vi "HFRR ADV v04 new software.vi"() -> ()   [LabVIEW 2025] (continued)
                n1292 = local write "FF 2"(0.0 ("FF 2")) -> ()
                n1293 = local write "reinit"(TRUE ("reinit")) -> ()
              }
            }
            n1294 = Select(t=0.0, s=w1593, f=w1592) -> (s? t:f=w1583:dbl)
            "COF 2" <- w1583
            n1295 = local write "COF 3"(w1583) -> ()
          }
        }
      }
    }
    n1296 = Wait (ms)(milliseconds to wait=u32 50) -> ()  [unwired: 1 out]
    n1297 = local read "Quit"() -> (w1521:bool)
    "Rate" <- 2500.0 ("No of Samples")
  }
  n1298 = while {
    tunnel: w57 -> [_]
    tunnel: [w1633] -> _
    tunnel: [w1609] -> w56
    i -> [w1633]
    stop <- w1609 stop-if-true
    # "C:\\LAB-IQ-NXT\\Scar View.exe"
    n1299 = local read "OK Button 16"() -> (w1622:bool)
    n1300 = local read "Main Tab"() -> (w1615:T2)
    n1301 = local read "service 3"() -> (w1616:bool)
    n1302 = local read "OPEN 6"() -> (w1618:bool)
    n1303 = local read "EDIT 2"() -> (w1620:bool)
    n1304 = flat-sequence {
      frame #0 {
        n1305 = local read "SAVE 2"() -> (w2235:bool)
        n1306 = stacked-sequence {
          frame #0 {
            n1307 = local read "EDIT"() -> (w2289:bool)
            n1308 = case shown="True" w2289 {
              tunnel: [u8 2 ("Disabled") u8 0 ("Disabled")] -> _
              frame False {
                w2291 = FALSE
                n1309 = local write "Password"("") -> ()
                n1310 = property on="SrvM CP" class="Bool (strict)"("Visible"=w2291) -> ()  [unwired: 2 in, 2 out]
                n1311 = property on="message" class="Str"("Visible"=w2291) -> ()  [unwired: 2 in, 2 out]
                n1312 = local write "x = y?"(w2291) -> ()
                n1313 = property on="Password" class="Str"("Visible"=w2291) -> ()  [unwired: 2 in, 2 out]
                n1314 = property on="ENTER THE NEW PASSWORD" class="Str"("Visible"=w2291) -> ()  [unwired: 2 in, 2 out]
                n1315 = property on="ENTER CURRENT PASSWORD" class="Str"("Visible"=w2291) -> ()  [unwired: 2 in, 2 out]
                n1316 = local write "SrvM CP"(w2291) -> ()
              }
              frame True {
                w2294 = TRUE
                n1317 = property on="SrvM CP" class="Bool (strict)"("Visible"=w2294) -> ()  [unwired: 2 in, 2 out]
                n1318 = property on="Password" class="Str"("Visible"=w2294) -> ()  [unwired: 2 in, 2 out]
              }
            }
            "dipl pwd" <- "@143$\n" ("dipl pwd")
          }
          frame #1 {
            # "Gain password"
            n1319 = String To Byte Array(string="ENTER CURRENT PASSWORD") -> (unsigned byte array=w2299:u8[])
            n1320 = Search 1D Array(1D array=w2299, element=u8 10) -> (index of element=w2302:i32)  [unwired: 1 in]
            n1321 = Index Array(array=w2299, index=w2302) -> (element=w2298:u8)
            n1322 = Equal?(x=w2298, y=10) -> (x = y?=w2296:bool)
            n1323 = case shown="True" w2296 {
              frame False {
                n1324 = property on="ENTER THE NEW PASSWORD" class="Str"("Visible"=FALSE) -> ()  [unwired: 2 in, 2 out]
              }
              frame True {
                # "password"
                # "change password logic"
                n1325 = local read "ENTER CURRENT PASSWORD"() -> (w2315:string)
                n1326 = local read "dipl pwd"() -> (w2309:string)
                n1327 = String To Byte Array(string=w2315) -> (unsigned byte array=w2317:u8[])
                n1328 = String To Byte Array(string=w2309) -> (unsigned byte array=w2310:u8[])
                n1329 = Array Size(array=w2317) -> (size(s)=w2314:i32)
                n1330 = Array Size(array=w2310) -> (size(s)=w2312:i32)
                n1331 = for {
                  N: w2314 -> [_]
                  tunnel: w2317 -> [w2341]
                  tunnel: [w2339] -> w2318 mode=indexing
                  tunnel: w2314 -> [w2333]
                  i -> [w2334]
                  n1332 = Decrement(x=w2333) -> (x-1=w2331:i32)
                  n1333 = Equal?(x=w2334, y=w2331) -> (x = y?=w2332:bool)
                  n1334 = Index Array(array=w2341, index=w2334) -> (element=w2335:u8)
                  n1335 = Number To Decimal String(number=w2335) -> (decimal integer string=w2340:string)  [unwired: 1 in]
                  n1336 = Select(t="", s=w2332, f="\r") -> (s? t:f=w2337:string)
                  n1337 = Concatenate Strings(w2340, w2337) -> (w2339:string)
                }
                n1338 = for {
                  N: w2312 -> [_]
                  tunnel: w2310 -> [w2329]
                  tunnel: [w2327] -> w2311 mode=indexing
                  tunnel: w2312 -> [w2324]
                  i -> [w2325]
                  n1339 = Decrement(x=w2324) -> (x-1=w2323:i32)
                  n1340 = Equal?(x=w2325, y=w2323) -> (x = y?=w2322:bool)
                  n1341 = Index Array(array=w2329, index=w2325) -> (element=w2328:u8)
                  n1342 = Number To Decimal String(number=w2328) -> (decimal integer string=w2326:string)  [unwired: 1 in]
                  n1343 = Select(t="", s=w2322, f="\r") -> (s? t:f=w2319:string)
                  n1344 = Concatenate Strings(w2326, w2319) -> (w2327:string)
                }
                n1345 = local read "string"() -> (w2316:string)
                n1346 = Concatenate Strings(w2311) -> (w2305:string)
                n1347 = Concatenate Strings(w2316) -> (w2313:string)
                n1348 = Concatenate Strings(w2318) -> (w2306:string)
                n1349 = Equal?(x=w2306, y=w2313) -> (x = y?=w2308:bool)
                n1350 = Equal?(x=w2306, y=w2305) -> (x = y?=w2304:bool)
                n1351 = Or(x=w2308, y=w2304) -> (x .or. y?=w2307:bool)
                n1352 = case shown="True" w2307 {
                  frame False {
                  }
                  frame True {
                    n1353 = property on="ENTER THE NEW PASSWORD" class="Str"("Visible"=TRUE) -> ()  [unwired: 2 in, 2 out]
                  }
                }
              }
            }
          }
          frame #2 {
            n1354 = String To Byte Array(string="ENTER THE NEW PASSWORD") -> (unsigned byte array=w2344:u8[])
            n1355 = Search 1D Array(1D array=w2344, element=u8 10) -> (index of element=w2348:i32)  [unwired: 1 in]
            n1356 = Index Array(array=w2344, index=w2348) -> (element=w2346:u8)
            n1357 = Equal?(x=w2346, y=10) -> (x = y?=w2343:bool)
            n1358 = case shown="False" w2343 {
              frame False {
              }
              frame True {
                n1359 = local write "EDIT"(FALSE) -> ()
                n1360 = local write "SrvM CP"(FALSE) -> ()
                n1361 = local read "ENTER THE NEW PASSWORD"() -> (w2351:string)
                n1362 = String To Byte Array(string=w2351) -> (unsigned byte array=w2356:u8[])
                n1363 = Array Size(array=w2356) -> (size(s)=w2353:i32)
                n1364 = for {
                  N: w2353 -> [_]
                  tunnel: w2356 -> [w2369]
                  tunnel: [w2366] -> w2358 mode=indexing
                  tunnel: w2353 -> [w2361]
                  i -> [w2359]
                  n1365 = Decrement(x=w2361) -> (x-1=w2362:i32)
                  n1366 = Equal?(x=w2359, y=w2362) -> (x = y?=w2363:bool)
                  n1367 = Index Array(array=w2369, index=w2359) -> (element=w2368:u8)
                  n1368 = Number To Decimal String(number=w2368) -> (decimal integer string=w2367:string)  [unwired: 1 in]
                  n1369 = Select(t="", s=w2363, f="\r") -> (s? t:f=w2360:string)
                  n1370 = Concatenate Strings(w2367, w2360) -> (w2366:string)
                }
                n1371 = local read "file path"() -> (w2350:path)
                n1372 = Concatenate Strings(w2358) -> (w2352:string)
                n1373 = Delete(path (use dialog)=w2350) -> (deleted path=w2354:path)  [unwired: 4 in, 2 out]
                n1374 = call <vilib>:"Write Characters To File.vi"("append to file? (new file:F)"=FALSE, "character string"=w2352, "file path (dialog if empty)"=w2354) -> ()  [unwired: 2 in, 1 out]
              }
            }
          }
          frame #3 {
            n1375 = case shown="True" "SrvM CP" {
              frame False {
                w2372 = ""
                n1376 = local write "ENTER CURRENT PASSWORD"(w2372) -> ()
                n1377 = local write "ENTER THE NEW PASSWORD"(w2372) -> ()
                n1378 = property on="ENTER CURRENT PASSWORD" class="Str"("Visible"=FALSE) -> ()  [unwired: 2 in, 2 out]
              }
              frame True {
                n1379 = property on="ENTER THE NEW PASSWORD" class="Str"() -> ("Visible"=w2373:bool)  [unwired: 2 in, 2 out]
                n1380 = Not(x=w2373) -> (.not. x?=w2374:bool)
                n1381 = property on="ENTER CURRENT PASSWORD" class="Str"("Visible"=w2374) -> ()  [unwired: 2 in, 2 out]
              }
            }
          }
          frame #4 {
            n1382 = String To Byte Array(string="Password") -> (unsigned byte array=w2381:u8[])
            n1383 = Search 1D Array(1D array=w2381, element=u8 10) -> (index of element=w2379:i32)  [unwired: 1 in]
            n1384 = Index Array(array=w2381, index=w2379) -> (element=w2380:u8)
            n1385 = Equal?(x=w2380, y=10) -> (x = y?=w2376:bool)
            n1386 = case shown="True" w2376 {
              frame False {
              }
              frame True {
                # "password"
                # "password"
                n1387 = local read "Password"() -> (w2394:string)
                n1388 = String To Byte Array(string=w2394) -> (unsigned byte array=w2397:u8[])
                n1389 = String To Byte Array(string="@143$\n") -> (unsigned byte array=w2383:u8[])
                n1390 = Array Size(array=w2397) -> (size(s)=w2392:i32)
                n1391 = Array Size(array=w2383) -> (size(s)=w2388:i32)
                n1392 = for {
                  N: w2392 -> [_]
                  tunnel: w2397 -> [w2431]
                  tunnel: [w2429] -> w2398 mode=indexing
                  tunnel: w2392 -> [w2426]
                  i -> [w2427]
                  n1393 = Decrement(x=w2426) -> (x-1=w2425:i32)
                  n1394 = Index Array(array=w2431, index=w2427) -> (element=w2430:u8)
                  n1395 = Equal?(x=w2427, y=w2425) -> (x = y?=w2424:bool)
                  n1396 = Number To Decimal String(number=w2430) -> (decimal integer string=w2428:string)  [unwired: 1 in]
                  n1397 = Select(t="", s=w2424, f="\r") -> (s? t:f=w2421:string)
                  n1398 = Concatenate Strings(w2428, w2421) -> (w2429:string)
                }
                n1399 = for {
                  N: w2388 -> [_]
                  tunnel: w2383 -> [w2442]
                  tunnel: [w2440] -> w2386 mode=indexing
                  tunnel: w2388 -> [w2437]
                  i -> [w2438]
                  n1400 = Decrement(x=w2437) -> (x-1=w2436:i32)
                  n1401 = Index Array(array=w2442, index=w2438) -> (element=w2441:u8)
                  n1402 = Equal?(x=w2438, y=w2436) -> (x = y?=w2435:bool)
                  n1403 = Number To Decimal String(number=w2441) -> (decimal integer string=w2439:string)  [unwired: 1 in]
                  n1404 = Select(t="", s=w2435, f="\r") -> (s? t:f=w2432:string)
                  n1405 = Concatenate Strings(w2439, w2432) -> (w2440:string)
                }
                n1406 = local read "file path"() -> (w2382:path)
                n1407 = call <vilib>:"Read Characters From File.vi"("file path (dialog if empty)"=w2382) -> ("character string"=w2396:string)  [unwired: 5 in, 3 out]
                "string" <- w2396
                n1408 = flat-sequence {
                  tunnel: [w2399] -> w2393
                  frame #0 {
                    w2399 = ""
                    n1409 = local write "Password"(w2399) -> ()
                  }
                }
                n1410 = Concatenate Strings(w2386) -> (w2387:string)
                n1411 = Concatenate Strings(w2396) -> (w2395:string)
                n1412 = Concatenate Strings(w2398) -> (w2390:string)
                n1413 = Equal?(x=w2390, y=w2395) -> (x = y?=w2385:bool)
                n1414 = Equal?(x=w2390, y=w2387) -> (x = y?=w2391:bool)
                n1415 = Or(x=w2385, y=w2391) -> (x .or. y?=w2384:bool)
                "x = y?" <- w2384
                n1416 = case shown="True" w2384 {
                  selector: w2384 -> [w2401 _]
                  tunnel: w2393 -> [_ _]
                  frame False {
                    n1417 = And(x=w2401, y=TRUE ("Visible")) -> (x .and. y?=w2402:bool)
                    n1418 = property on="message" class="Str"("Visible"=w2402) -> ()  [unwired: 2 in, 2 out]
                  }
                  frame True {
                    n1419 = control-ref of="This VI"() -> (w2413:refnum<vi>)
                    n1420 = property class="VI"(reference=w2413) -> (reference out=w2404:refnum<vi>, error out=w2408:errorcluster, "Panel"=w2412:refnum<vi>)  [unwired: 1 in]
                    n1421 = property on="message" class="Str"("Visible"=FALSE) -> ()  [unwired: 2 in, 2 out]
                    n1422 = property class="Pnl"(reference=w2412, error in=w2408) -> (reference out=w2406:refnum<vi>, error out=w2409:errorcluster, "Panes[]"=w2411:refnum<vi>[])
                    n1423 = for {
                      tunnel: w2411 -> [w2420] mode=indexing
                      tunnel: T15."Always On" ("Horizontal Scrollbar Visibility") -> [w2419]
                      tunnel: w2409 -> [w2416]
                      tunnel: [w2415] -> w2407
                      n1424 = property class="Pane"(reference=w2420, error in=w2416, "HorizScrollbarVisibility"=w2419) -> (reference out=w2417:refnum<vi>, error out=w2418:errorcluster)
                      n1425 = Close Reference(reference=w2417, error in (no error)=w2418) -> (error out=w2415:errorcluster)
                    }
                    n1426 = Close Reference(reference=w2406, error in (no error)=w2407) -> (error out=w2405:errorcluster)
                    n1427 = Close Reference(reference=w2404, error in (no error)=w2405) -> (error out=→"error out 6":errorcluster)
                  }
                }
              }
            }
          }
        }
        n1428 = local read "x = y?"() -> (w2241:bool)
        n1429 = local read "HUMIDITY: 2"() -> (w2243:dbl)
        n1430 = local read "HUMIDITY:"() -> (w2242:dbl)
        n1431 = property on="Port 2 Error" class="Clust (strict)"("Visible"="EDIT") -> ()  [unwired: 2 in, 2 out]
        n1432 = property on="Port 1 Error" class="Clust (strict)"("Visible"="EDIT") -> ()  [unwired: 2 in, 2 out]
        n1433 = case shown="True" "SrvM CP 2" {
          frame False {
          }
          frame True {
            n1434 = local write "SrvM CP 2"(FALSE ("SrvM CP 2")) -> ()
            n1435 = local read "HUMIDITY: 2"() -> (w2282:dbl)
            n1436 = local read "TEMP INTERCEPT: 2"() -> (w2281:dbl)
            n1437 = local read "DISPLACEMENT : 4"() -> (w2285:dbl)
            n1438 = local read "TEMPERATURE : 2"() -> (w2284:dbl)
            n1439 = local read "STROKE GAIN : 2"() -> (w2286:dbl)
            n1440 = local read "FRIC. FORCE : 2"() -> (w2287:dbl)
            n1441 = local read "AIR TEMP INTERCEPT: 2"() -> (w2280:dbl)
            n1442 = local read "AIR TEMPERATURE : 2"() -> (w2283:dbl)
            n1443 = local write "HUMIDITY:"(w2282) -> ()
            n1444 = local write "AIR TEMP INTERCEPT:"(w2281) -> ()
            n1445 = local write "TEMPERATURE :"(w2284) -> ()
            n1446 = local write "FRIC. FORCE :"(w2287) -> ()
            n1447 = local write "STROKE GAIN :"(w2286) -> ()
            n1448 = local write "DISPLACEMENT :"(w2285) -> ()
            n1449 = local write "AIR TEMPERATURE :"(w2283) -> ()
            n1450 = local write "TEMP INTERCEPT:"(w2280) -> ()
          }
        }
        n1451 = Or(x="SAVE", y=w2235) -> (x .or. y?=w2236:bool)
        n1452 = And(x="EDIT", y=w2241) -> (x .and. y?=w2239:bool)
        n1453 = local read "DISPLACEMENT : 4"() -> (w2252:dbl)
        n1454 = local read "TEMPERATURE : 2"() -> (w2250:dbl)
        n1455 = local read "STROKE GAIN : 2"() -> (w2256:dbl)
        n1456 = local read "DISPLACEMENT :"() -> (w2251:dbl)
        n1457 = local read "FRIC. FORCE : 2"() -> (w2259:dbl)
        n1458 = local read "TEMPERATURE :"() -> (w2248:dbl)
        n1459 = local read "STROKE GAIN :"() -> (w2255:dbl)
        n1460 = local read "FRIC. FORCE :"() -> (w2258:dbl)
        n1461 = case shown="True" w2239 {
          tunnel: [u8 2 ("Disabled") u8 0 ("Disabled")] -> w2238
          tunnel: [w2603 TRUE ("Visible")] -> w2237
          frame False {
            w2603 = FALSE ("Visible")
            n1462 = local write "EDIT 2"(w2603) -> ()
          }
          frame True {
          }
        }
        n1463 = case shown="True" w2236 {
          frame False {
          }
          frame True {
            n1464 = stacked-sequence {
              seq-local: [w2451 _ _] -> [_ w2598 _]
              frame #0 {
                (unwired) i16 5 ("precision (6)")
                # "[CH1]    - FF\n[CH2]   - TEMPERATURE\n[CH3]    - Humidity\n[CH4]    - AIR TEMP\n[CH5]\\- Visa Uno\n[CH6] \\- Visa Due\n[CH7]  \\- file path\n[CH8]   - Displacement Gain\n[CHA]   - Stroke Gain\n[CHB]   - Stroke PID Gain\n[CHC]   -Language Selection\n[CHD]   -Power +\n[CHE]   -Power_\n[CHF]   -Heater\n[CHG]   -Humidity Wet\n[CHH]   -Humidity Dry\n[CHI]   -Integral Time"
                n1465 = local read "Language Selection"() -> (w2499:enum16{"English", "Russian"})
                n1466 = local read "CH-HUMIDITY WET"() -> (w2457:u16)
                n1467 = local read "CH-HUMIDITY DRY"() -> (w2454:u16)
                n1468 = local read "STROKE GAIN :"() -> (w2443:dbl)
                n1469 = local read "CH-POWER +"() -> (w2466:u16)
                n1470 = local read "CH-POWER -"() -> (w2463:u16)
                n1471 = local read "CH-HEATER"() -> (w2460:u16)
                n1472 = local read "AIR TEMPERATURE :"() -> (w2446:dbl)
                n1473 = local read "DISPLACEMENT :"() -> (w2444:dbl)
                n1474 = local read "TEMPERATURE :"() -> (w2447:dbl)
                n1475 = local read "FRIC. FORCE :"() -> (w2448:dbl)
                n1476 = local read "HUMIDITY:"() -> (w2445:dbl)
                n1477 = Path To String(path="File Path") -> (string=w2515:string)
                n1478 = Number To Fractional String(number=w2443, width (-)=i16 10 ("precision (6)"), precision (6)=i16 5) -> (F-format string=w2506:string)  [unwired: 1 in]
                n1479 = Number To Fractional String(number=w2499, width (-)=i16 10 ("precision (6)"), precision (6)=i16 5) -> (F-format string=w2495:string)  [unwired: 1 in]
                n1480 = Number To Fractional String(number=w2466, width (-)=i16 10 ("precision (6)"), precision (6)=i16 5) -> (F-format string=w2489:string)  [unwired: 1 in]
                n1481 = Number To Fractional String(number=w2463, width (-)=i16 10 ("precision (6)"), precision (6)=i16 5) -> (F-format string=w2486:string)  [unwired: 1 in]
                n1482 = Number To Fractional String(number=w2460, width (-)=i16 10 ("precision (6)"), precision (6)=i16 5) -> (F-format string=w2481:string)  [unwired: 1 in]
                n1483 = Number To Fractional String(number=w2457, width (-)=i16 10 ("precision (6)"), precision (6)=i16 5) -> (F-format string=w2478:string)  [unwired: 1 in]
                n1484 = Number To Fractional String(number=w2454, width (-)=i16 10 ("precision (6)"), precision (6)=i16 5) -> (F-format string=w2473:string)  [unwired: 1 in]
                n1485 = local read "Com Port 1"() -> (w2450:refnum<visa-resource-name>)
                n1486 = local read "Com Port 2"() -> (w2449:refnum<visa-resource-name>)
                n1487 = Concatenate Strings(w2515, "\\" ("string")) -> (w2514:string)
                n1488 = Number To Fractional String(number=w2448, width (-)=i16 10 ("precision (6)"), precision (6)=i16 5) -> (F-format string=w2547:string)  [unwired: 1 in]
                n1489 = Number To Fractional String(number=w2447, width (-)=i16 10 ("precision (6)"), precision (6)=i16 5) -> (F-format string=w2546:string)  [unwired: 1 in]
                n1490 = Number To Fractional String(number=w2445, width (-)=i16 10 ("precision (6)"), precision (6)=i16 5) -> (F-format string=w2540:string)  [unwired: 1 in]
                n1491 = Number To Fractional String(number=w2446, width (-)=i16 10 ("precision (6)"), precision (6)=i16 5) -> (F-format string=w2534:string)  [unwired: 1 in]
                n1492 = Number To Fractional String(number=w2444, width (-)=i16 10 ("precision (6)"), precision (6)=i16 5) -> (F-format string=w2507:string)  [unwired: 1 in]
                n1493 = Concatenate Strings("[CHA]" ("string"), w2506, "- Stroke Gain" ("string"), "\r") -> (w2500:string)
                n1494 = Concatenate Strings("[CHC]" ("string"), w2495, "-Language Selection" ("string"), "\r") -> (w2492:string)
                n1495 = Concatenate Strings("[CHD]" ("string"), w2489, "-Power +" ("string"), "\r") -> (w2471:string)
                n1496 = Concatenate Strings("[CHG]" ("string"), w2478, "-Humidity Wet" ("string"), "\r") -> (w2468:string)
                n1497 = Concatenate Strings("[CHH]" ("string"), w2473, "-Humidity Dry" ("string"), "\r") -> (w2467:string)
                n1498 = Concatenate Strings("[CH1]" ("string"), w2547, " - FF" ("string"), "\r") -> (w2545:string)
                n1499 = Concatenate Strings("[CH2]" ("string"), w2546, " - TEMPERATURE" ("string"), "\r") -> (w2544:string)
                n1500 = Concatenate Strings("[CH3]" ("string"), w2540, " - Humidity" ("string"), "\r") -> (w2537:string)
                n1501 = Concatenate Strings("[CH4]" ("string"), w2534, " - AIR TEMP" ("string"), "\r") -> (w2530:string)
                n1502 = Concatenate Strings("[CH5]" ("string"), w2450, "- Visa Uno" ("string"), "\r") -> (w2523:string)
                n1503 = Concatenate Strings("[CH6]" ("string"), w2449, "- Visa Due" ("string"), "\r") -> (w2518:string)
                n1504 = Concatenate Strings("[CH7]" ("string"), w2514, "- file path" ("string"), "\r") -> (w2517:string)
                n1505 = Concatenate Strings("[CH8]" ("string"), w2507, "- Displacement Gain" ("string"), "\r") -> (w2510:string)
                n1506 = Concatenate Strings("[CHE]" ("string"), w2486, "-Power_" ("string"), "\r") -> (w2470:string)
                n1507 = Concatenate Strings("[CHF]" ("string"), w2481, "-Heater" ("string"), "\r") -> (w2469:string)
                n1508 = Concatenate Strings(w2545, w2544, w2537, w2530, w2523, w2518, w2517, w2510, w2500, w2492, w2471, w2470, w2469, w2468, w2467) -> (w2451:string)
                "gain" <- w2451
              }
              frame #1 {
                n1509 = local read "Camera Port :"() -> (w2559:string)
                n1510 = local read "C3 :"() -> (w2567:refnum<visa-resource-name>)
                n1511 = local read "TEMP INTERCEPT:"() -> (w2568:dbl)
                n1512 = local read "AIR TEMP INTERCEPT:"() -> (w2569:dbl)
                n1513 = Concatenate Strings("[CH8]" ("string"), w2559, "- Visa Camera" ("string"), "\r") -> (w2558:string)
                n1514 = Concatenate Strings("[CH7]" ("string"), w2567, "- Visa Humidity" ("string"), "\r") -> (w2563:string)
                n1515 = Number To Fractional String(number=w2568, width (-)=i16 10 ("precision (6)"), precision (6)=i16 5) -> (F-format string=w2586:string)  [unwired: 1 in]
                n1516 = local read "Com Port 3"() -> (w2570:refnum<visa-resource-name>)
                n1517 = Number To Fractional String(number=w2569, width (-)=i16 10 ("precision (6)"), precision (6)=i16 5) -> (F-format string=w2593:string)  [unwired: 1 in]
                n1518 = Concatenate Strings("[CHK]" ("string"), w2586, "-TEMP INTERCEPT" ("string"), "\r") -> (w2582:string)
                n1519 = Concatenate Strings("[SNO]" ("string"), "S.NO", "-" ("string"), "\r") -> (w2578:string)
                n1520 = Concatenate Strings("[CHJ]" ("string"), w2593, "-AIR TEMP INTERCEPT" ("string"), "\r") -> (w2583:string)
                n1521 = Concatenate Strings("[CHL]" ("string"), w2570, "- Visa humid" ("string"), "\r") -> (w2573:string)
                n1522 = String To Path(string="C:\\LAB-IQ\\calibrate WO 2465.dcf") -> (path=w2571:path)
                n1523 = Concatenate Strings(w2598, w2583, w2582, w2578, w2573, w2563, w2558) -> (w2597:string)
                n1524 = call <vilib>:"Write Characters To File.vi"("append to file? (new file:F)"=FALSE, "character string"=w2597, "file path (dialog if empty)"=w2571) -> ()  [unwired: 2 in, 1 out]
              }
              frame #2 {
                n1525 = local write "Lan flag"(0.0 ("Lan flag")) -> ()
                n1526 = local write "conststatus"(0.0 ("rpm value : 2")) -> ()
                n1527 = local write "SAVE"(FALSE ("OK Button 14")) -> ()
                n1528 = local write "SAVE 2"(FALSE ("SAVE 2")) -> ()
              }
            }
          }
        }
        n1529 = Subtract(x=w2243, y=w2242) -> (x-y=w2244:dbl)
        n1530 = local read "AIR TEMPERATURE : 2"() -> (w2247:dbl)
        n1531 = local read "AIR TEMPERATURE :"() -> (w2246:dbl)
        n1532 = Divide(x=w2244, y=w2242) -> (x/y=w2266:dbl)
        n1533 = Subtract(x=w2259, y=w2258) -> (x-y=w2257:dbl)
        n1534 = Subtract(x=w2250, y=w2248) -> (x-y=w2249:dbl)
        n1535 = Subtract(x=w2256, y=w2255) -> (x-y=w2254:dbl)
        n1536 = Subtract(x=w2252, y=w2251) -> (x-y=w2253:dbl)
        n1537 = Subtract(x=w2247, y=w2246) -> (x-y=w2245:dbl)
        n1538 = Divide(x=w2257, y=w2258) -> (x/y=w2277:dbl)
        n1539 = Divide(x=w2249, y=w2248) -> (x/y=w2270:dbl)
        n1540 = Divide(x=w2254, y=w2255) -> (x/y=w2274:dbl)
        n1541 = Divide(x=w2253, y=w2251) -> (x/y=w2273:dbl)
        n1542 = Multiply(x=w2266, y=100.0) -> (x*y=→"HUMIDITY  Calibration Error":dbl)
        n1543 = Divide(x=w2245, y=w2246) -> (x/y=w2269:dbl)
        n1544 = Multiply(x=w2277, y=100.0) -> (x*y=→"FRIC. FORCE Calibration Error":dbl)
        n1545 = Multiply(x=w2270, y=100.0) -> (x*y=→"TEMPERATURE  Calibration Error":dbl)
        n1546 = Multiply(x=w2274, y=100.0) -> (x*y=→"STROKE Calibration Error":dbl)
        n1547 = Multiply(x=w2273, y=100.0) -> (x*y=→"DISPLACEMENT  Calibration Error":dbl)
        n1548 = property on="EDIT 2" class="Bool (strict)"("Visible"=w2237) -> ()  [unwired: 2 in, 2 out]
        n1549 = property on="SAVE" class="Bool (strict)"("Visible"=w2237) -> ()  [unwired: 2 in, 2 out]
        n1550 = property on="SrvM CP" class="Bool (strict)"("Disabled"=w2238) -> ()  [unwired: 2 in, 2 out]
        n1551 = property on="visa due" class="CmbBox"("Disabled"=w2238) -> ()  [unwired: 2 in, 2 out]
        n1552 = property on="File Path" class="Path"("Disabled"=w2238) -> ()  [unwired: 2 in, 2 out]
        n1553 = Multiply(x=w2269, y=100.0) -> (x*y=→"AIR TEMPERATURE  Calibration Error":dbl)
        n1554 = property on="Language Selection" class="Enum (strict)"("Visible"=w2237) -> ()  [unwired: 2 in, 2 out]
        n1555 = property on="Tab Control 7" class="TabCtl (strict)"("Disabled"=w2238) -> ()  [unwired: 2 in, 2 out]
        n1556 = property on="AIR TEMP INTERCEPT:" class="DigNum (strict)"("Disabled"=w2238) -> ()  [unwired: 2 in, 2 out]
        n1557 = property on="CH-POWER -" class="DigNum (strict)"("Disabled"=w2238) -> ()  [unwired: 2 in, 2 out]
        n1558 = property on="CH-POWER +" class="DigNum (strict)"("Disabled"=w2238) -> ()  [unwired: 2 in, 2 out]
        n1559 = property on="AIR TEMPERATURE :" class="DigNum (strict)"("Disabled"=w2238) -> ()  [unwired: 2 in, 2 out]
        n1560 = property on="STROKE GAIN :" class="DigNum (strict)"("Disabled"=w2238) -> ()  [unwired: 2 in, 2 out]
        n1561 = property on="SPEED OUT:" class="DigNum (strict)"("Disabled"=w2238) -> ()  [unwired: 2 in, 2 out]
        n1562 = property on="CH-HUMIDITY DRY" class="DigNum (strict)"("Disabled"=w2238) -> ()  [unwired: 2 in, 2 out]
        n1563 = property on="HUMIDITY:" class="DigNum (strict)"("Disabled"=w2238) -> ()  [unwired: 2 in, 2 out]
        n1564 = property on="CH-HUMIDITY WET" class="DigNum (strict)"("Disabled"=w2238) -> ()  [unwired: 2 in, 2 out]
        n1565 = property on="TEMPERATURE :" class="DigNum (strict)"("Disabled"=w2238) -> ()  [unwired: 2 in, 2 out]
        n1566 = property on="DISPLACEMENT :" class="DigNum (strict)"("Disabled"=w2238) -> ()  [unwired: 2 in, 2 out]
        n1567 = property on="CH-HEATER" class="DigNum (strict)"("Disabled"=w2238) -> ()  [unwired: 2 in, 2 out]
        n1568 = property on="TEMP INTERCEPT:" class="DigNum (strict)"("Disabled"=w2238) -> ()  [unwired: 2 in, 2 out]
        n1569 = property on="FRIC. FORCE :" class="DigNum (strict)"("Disabled"=w2238) -> ()  [unwired: 2 in, 2 out]
      }
    }
    n1570 = local read "RUN"() -> (w1632:bool)
    n1571 = local read "RUN"() -> (w1630:bool)
    n1572 = disable-structure shown="Disabled" {
      disable-tunnel: [w1647 _] -> w1613
      disable-tunnel: [w1646 _] -> w1611
      frame Disabled {
        n1573 = local read "Temperature before test"() -> (w1640:dbl)
        n1574 = local read "Temperature after test"() -> (w1653:dbl)
        n1575 = case shown="True" "Save Results" {
          frame False {
          }
          frame True {
            w1669 = "\r"
            n1576 = local write "Save Results"(FALSE ("OK Button 5")) -> ()
            n1577 = local read "Temperature before test"() -> (w1707:dbl)
            n1578 = local read "Temperature after test"() -> (w1709:dbl)
            n1579 = local read "Humidity before test"() -> (w1706:dbl)
            n1580 = local read "Humidity after test"() -> (w1708:dbl)
            n1581 = local read "WS1.4"() -> (w1713:dbl)
            n1582 = local read "AVP"() -> (w1711:dbl)
            n1583 = Number To Fractional String(number=w1713, width (-)=i16 6, precision (6)=i16 1) -> (F-format string=w1673:string)  [unwired: 1 in]
            n1584 = local read "MWSD"() -> (w1710:dbl)
            n1585 = local read "String"() -> (w1702:string)
            n1586 = local read "FILE"() -> (w1705:string)
            n1587 = local read "HCF"() -> (w1712:dbl)
            n1588 = Number To Fractional String(number=w1706, width (-)=i16 6, precision (6)=i16 1) -> (F-format string=w1698:string)  [unwired: 1 in]
            n1589 = Number To Fractional String(number=w1707, width (-)=i16 6, precision (6)=i16 1) -> (F-format string=w1695:string)  [unwired: 1 in]
            n1590 = Number To Fractional String(number=w1708, width (-)=i16 6, precision (6)=i16 1) -> (F-format string=w1691:string)  [unwired: 1 in]
            n1591 = Number To Fractional String(number=w1709, width (-)=i16 6, precision (6)=i16 1) -> (F-format string=w1687:string)  [unwired: 1 in]
            n1592 = Number To Fractional String(number=w1711, width (-)=i16 6, precision (6)=i16 3) -> (F-format string=w1680:string)  [unwired: 1 in]
            n1593 = Concatenate Strings(w1702, w1705) -> (w1724:string)
            n1594 = Number To Fractional String(number=w1710, width (-)=i16 6, precision (6)=i16 1) -> (F-format string=w1684:string)  [unwired: 1 in]
            n1595 = Number To Fractional String(number=w1712, width (-)=i16 6, precision (6)=i16 2) -> (F-format string=w1678:string)  [unwired: 1 in]
            n1596 = Concatenate Strings("(" ("string"), w1673, ")Microns" ("string")) -> (w1672:string)
            n1597 = local read "REMARKS"() -> (w1704:string)
            "REMARKS 2" <- w1704
            n1598 = Concatenate Strings("(" ("string"), w1698, " ) % RH," ("string")) -> (w1699:string)
            n1599 = Concatenate Strings(w1678, ")" ("string")) -> (w1676:string)
            n1600 = Concatenate Strings("(" ("string"), w1695, ")  Deg C ," ("string")) -> (w1694:string)
            n1601 = Concatenate Strings("(" ("string"), w1691, " ) % RH," ("string")) -> (w1690:string)
            n1602 = Concatenate Strings("(" ("string"), w1687, ")  Deg C ," ("string")) -> (w1686:string)
            n1603 = Concatenate Strings("(" ("string"), w1684, ")  Microns," ("string")) -> (w1683:string)
            n1604 = Concatenate Strings("(" ("string"), w1680, ")  kPa," ("string")) -> (w1670:string)
            n1605 = Concatenate Strings(w1724, ".dwm" ("Substring")) -> (w1722:string)
            n1606 = String To Path(string=w1722) -> (path=w1721:path)
            n1607 = Concatenate Strings(w1704, w1669, " Humidity before test= " ("Substring"), w1699, w1669, " Temperature before test = " ("Substring"), w1694, w1669, " Humidity after test= " ("Substring"), w1690, w1669, "Temperature after test = " ("Substring"), w1686, w1669, "MSD = " ("Substring"), w1683, w1669, "  AVP = " ("Substring"), w1670, w1669, "  HCF                     =( " ("Substring"), w1676, w1669, " WS1.4                  = " ("Substring"), w1672, w1669) -> (w1668:string)
            "data" <- w1668
            n1608 = call <vilib>:"Write Characters To File.vi"("append to file? (new file:F)"=FALSE, "character string"=w1668, "file path (dialog if empty)"=w1721) -> ()  [unwired: 2 in, 1 out]
            n1609 = Match Pattern(string=w1668, regular expression="!") -> (after substring=→"export":string)  [unwired: 1 in, 3 out]
          }
        }
        n1610 = Add(x=231.864, y=w1640) -> (x+y=w1637:dbl)
        n1611 = Add(x=231.864, y=w1653) -> (x+y=w1650:dbl)
        n1612 = Divide(x=1705.984, y=w1637) -> (x/y=w1638:dbl)
        n1613 = Divide(x=1705.984, y=w1650) -> (x/y=w1651:dbl)
        n1614 = local read "Humidity before test"() -> (w1642:dbl)
        n1615 = local read "Humidity after test"() -> (w1655:dbl)
        n1616 = Subtract(x=8.017352 ("y"), y=w1638) -> (x-y=w1664:dbl)
        n1617 = Subtract(x=8.017352 ("y"), y=w1651) -> (x-y=w1658:dbl)
        n1618 = expression code="10**y"(w1664) -> (w1644:dbl)
        n1619 = expression code="10**y"(w1658) -> (w1657:dbl)
        n1620 = Multiply(x=w1642, y=w1644) -> (x*y=w1643:dbl)
        n1621 = Multiply(x=w1655, y=w1657) -> (x*y=w1656:dbl)
        n1622 = Divide(x=w1643, y=750.0) -> (x/y=w1659:dbl)
        n1623 = Divide(x=w1656, y=750.0) -> (x/y=w1660:dbl)
        n1624 = Add(x=w1659, y=w1660) -> (x+y=w1661:dbl)
        n1625 = Divide(x=w1661, y=2.0) -> (x/y=w1663:dbl)
        n1626 = local write "AVP"(w1663) -> ()
        n1627 = Subtract(x=1.4, y=w1663) -> (x-y=w1646:dbl)
        n1628 = local read "HCF"() -> (w1647:dbl)
      }
      frame Enabled {
      }
    }
    n1629 = case shown="True" "EDIT 3" {
      frame False {
      }
      frame True {
        n1630 = local write "EDIT 3"(FALSE ("EDIT 3")) -> ()
        n1631 = local write "Main Tab"(T2."About" ("Main Tab")) -> ()
      }
    }
    n1632 = case shown="False" w1632 {
      frame False {
        n1633 = local read "stopT"() -> (w2610:bool)
        n1634 = case shown="True" w2610 {
          frame False {
          }
          frame True {
            n1635 = local write "stopT"(FALSE) -> ()
          }
        }
      }
      frame True {
        "stopT" <- TRUE
      }
    }
    n1636 = case shown="False" w1630 {
      frame False {
      }
      frame True {
      }
    }
    n1637 = case shown="True" w1620 {
      frame False {
        n1638 = property on="Password 2" class="Str"("Visible"=FALSE) -> ()  [unwired: 2 in, 2 out]
        n1639 = local write "Password 2"("" ("Password")) -> ()
      }
      frame True {
        n1640 = property on="Password 2" class="Str"("Visible"=TRUE) -> ()  [unwired: 2 in, 2 out]
        n1641 = Equal?(x="Password 2", y="HFRR1234") -> (x = y?=w1752:bool)
        n1642 = case shown="True" w1752 {
          tunnel: "Password 2" -> [w1755 _]
          frame False {
            n1643 = String Length(string=w1755) -> (length=w1756:i32)
            n1644 = Greater Than 0?(x=w1756) -> (x > 0?=w1754:bool)
            n1645 = case shown="False" w1754 {
              frame False {
                n1646 = property on="Password 2" class="Str"("Caption.Text"="Password (Advance Setting)") -> ()  [unwired: 2 in, 2 out]
              }
              frame True {
                n1647 = property on="Password 2" class="Str"("Caption.Text"="Incorrect Password!") -> ()  [unwired: 2 in, 2 out]
              }
            }
          }
          frame True {
            n1648 = local write "EDIT 2"(FALSE ("EDIT 2")) -> ()
            n1649 = local write "Password 2"("" ("Password")) -> ()
            n1650 = local write "Main Tab"(T2."Advance" ("Main Tab")) -> ()
            n1651 = local write "Main Dashboard Buttons"(T1."Advance" ("Main Dashboard Buttons")) -> ()
          }
        }
      }
    }
    n1652 = case shown="True" "Prog Uno" {
      frame False {
      }
      frame True {
        n1653 = stacked-sequence {
          frame #0 {
            n1654 = Delete(path (use dialog)=path "C:/LAB-IQ-NXT/UNOCOMPILE.bat" ("working directory")) -> ()  [unwired: 4 in, 3 out]
          }
          frame #1 {
            n1655 = local read "Com Port 1"() -> (w2217:refnum<visa-resource-name>)
            n1656 = Concatenate Strings("cmd.exe /c \"mode " ("command line"), w2217, ":1200,n,8,1\"\n" ("command line")) -> (w2222:string)
            n1657 = Concatenate Strings(w2222, "CD\\\nCD WinDucom\navrdude -C avrdude.conf -v -patmega328p -carduino -P" ("command line"), w2217, " -b115200 -D -Uflash:w:UNO_V20.hex:i\n" ("command line"), "\r") -> (w2224:string)
            "STR" <- w2224
            n1658 = call <vilib>:"Write Characters To File.vi"("append to file? (new file:F)"=FALSE, "character string"=w2224, "file path (dialog if empty)"=path "C:/LAB-IQ/UNOCOMPILE.bat" ("working directory")) -> ()  [unwired: 2 in, 1 out]
          }
          frame #2 {
            n1659 = disable-structure shown="Disabled" {
              frame Disabled {
                w2228 = "cmd.exe  /c \"C:\\LAB-IQ-NXT\\UNOCOMPILE.bat\"" ("string")
                n1660 = local write "Prog Uno"(FALSE ("run minimized? (F)")) -> ()
                n1661 = call <vilib>:"System Exec.vi"("expected output size  (4096)"=u32 65535, "run minimized? (F)"=FALSE, "wait until completion? (T)"=TRUE ("run minimized? (F)"), "working directory"=path "C:/LAB-IQ-NXT", "standard input"=w2228, "command line"=w2228) -> ("error out"=w2227:errorcluster, "standard output"=→"String 42":string)  [unwired: 2 in, 2 out]
                "error out 3" <- w2227
                n1662 = flat-sequence {
                  tunnel: w2227 -> [_]
                  frame #0 {
                  }
                }
              }
              frame Enabled {
              }
            }
          }
        }
      }
    }
    n1663 = case shown="\"CEC F-096-A-06\"" "TEST STANDARD" {
      tunnel: [2.0 ("Set Temp") 0.0 ("Set Temp") 2.0 ("Set Temp") 0.0 ("Set Temp")] -> w1621
      frame "ASTM D6079", Default {
        w2174 = 50.0 ("Hz")
        w2175 = 53.0 ("Set Rh")
        w2177 = 1.0 ("Set Strk")
        w2176 = 60.0 ("Set Temp")
        # "astm hide"
        n1664 = local write "NORMAL LOAD"(200.0 ("NORMAL LOAD")) -> ()
        n1665 = local write "Set Strk"(w2177) -> ()
        n1666 = local write "Set Hz"(w2174) -> ()
        n1667 = local write "Set Temp"(w2176) -> ()
        n1668 = local write "Set Rh"(w2175) -> ()
        n1669 = local write "test time"(75.0 ("test time")) -> ()
        n1670 = local write "Set Stroke:"(w2177) -> ()
        n1671 = local write "Set Humidity:"(w2175) -> ()
        n1672 = local write "Set Frequency:"(w2174) -> ()
        n1673 = local write "Set Temperature:"(w2176) -> ()
        "Test Standard" <- "ASTM D6079" ("Test Standard 2")
      }
      frame "ISO 12156" {
        n1674 = local write "Set Strk"(1.0 ("Set Strk")) -> ()
        n1675 = local write "NORMAL LOAD"(200.0 ("NORMAL LOAD")) -> ()
        n1676 = local write "Set Temp"(60.0 ("Set Temp")) -> ()
        n1677 = local write "test time"(75.0 ("test time")) -> ()
        n1678 = local write "Set Hz"(50.0 ("Hz")) -> ()
        n1679 = local write "Set Rh"(53.0 ("Set Rh")) -> ()
      }
      frame "CEC F-096-A-06" {
        n1680 = local write "Set Strk"(1.0 ("Set Strk")) -> ()
        n1681 = local write "NORMAL LOAD"(200.0 ("NORMAL LOAD")) -> ()
        n1682 = local write "Set Temp"(60.0 ("Set Temp")) -> ()
        n1683 = local write "test time"(75.0 ("test time")) -> ()
        n1684 = local write "Set Hz"(50.0 ("Hz")) -> ()
        n1685 = local write "Set Rh"(53.0 ("Set Rh")) -> ()
      }
      frame "Custom" {
      }
    }
    n1686 = case shown="True" "Prog Due" {
      frame False {
      }
      frame True {
        n1687 = stacked-sequence {
          frame #0 {
            n1688 = Delete(path (use dialog)=path "C:/LAB-IQ/DUECOMPILE.bat" ("working directory")) -> ()  [unwired: 4 in, 3 out]
          }
          frame #1 {
            n1689 = disable-structure shown="Disabled" {
              frame Disabled {
                n1690 = local read "visa due"() -> (w2199:string)
                n1691 = Concatenate Strings("cmd.exe /c \"mode " ("command line"), w2199, ":1200,n,8,1\"\n" ("command line")) -> (w2204:string)
                n1692 = Concatenate Strings(w2204, "CD\\\nCD WinDucom\nTIMEOUT 1\n bossac.exe -i -d --port=" ("command line"), w2199, " -U false -e -w -v -b DUE.bin -R\n" ("command line"), "\r") -> (w2206:string)
                "concatenated string 2" <- w2206
                n1693 = call <vilib>:"Write Characters To File.vi"("append to file? (new file:F)"=FALSE, "character string"=w2206, "file path (dialog if empty)"=path "C:/LAB-IQ-NXT/DUECOMPILE.bat" ("working directory")) -> ()  [unwired: 2 in, 1 out]
              }
              frame Enabled {
              }
            }
          }
          frame #2 {
            # "C:\\LAB-IQ-NXT\\DUECOMPILE.bat"
            n1694 = disable-structure shown="Disabled" {
              frame Disabled {
                w2211 = "cmd.exe  /c \"C:\\LAB-IQ-NXT\\DUECOMPILE.bat\"" ("string")
                n1695 = call <vilib>:"System Exec.vi"("expected output size  (4096)"=u32 65535, "run minimized? (F)"=FALSE, "wait until completion? (T)"=TRUE ("run minimized? (F)"), "working directory"=path "C:/LAB-IQ-NXT", "standard input"=w2211, "command line"=w2211) -> ("error out"=w2210:errorcluster, "standard output"=→"String 44":string)  [unwired: 2 in, 2 out]
                "error out 4" <- w2210
                n1696 = flat-sequence {
                  tunnel: w2210 -> [_]
                  frame #0 {
                  }
                }
              }
              frame Enabled {
              }
            }
            n1697 = local write "Prog Due"(FALSE ("Prog Due")) -> ()
          }
        }
      }
    }
    n1698 = Or(x=w1618, y=w1616) -> (x .or. y?=w1617:bool)
    n1699 = case shown="\"About\"" w1615 {
      tunnel: [T20."Acquire" ("Main Tab") T20."Compare Files" ("Main Tab") T20."About" ("Main Tab")] -> w1628
      frame "Acquire", Default {
      }
      frame "Compare Files" {
      }
      frame "About" {
      }
    }
    n1700 = Or(x=w1622, y="OPEN") -> (x .or. y?=w1623:bool)
    n1701 = case shown="True" w1623 {
      tunnel: w1622 -> [_ w1763]
      frame False {
      }
      frame True {
        n1702 = stacked-sequence {
          tunnel: w1763 -> [_ w1830 _ _]
          frame #0 {
            w1779 = "  " ("String 6")
            n1703 = local write "OPEN"(FALSE ("open")) -> ()
            n1704 = local read "string1 2"() -> (w1767:string)
            n1705 = local read "string1 3"() -> (w1766:string)
            n1706 = local read "string1 4"() -> (w1765:string)
            n1707 = property on="OPEN" class="Bool (strict)"("Visible"=FALSE) -> ()  [unwired: 2 in, 2 out]
            n1708 = local write "String 6"(w1779) -> ()
            n1709 = local write "String 7"(w1779) -> ()
            n1710 = local write "String 8"(w1779) -> ()
            n1711 = local write "String 12"(w1779) -> ()
            n1712 = local read "OK Button 16"() -> (w1764:bool)
            n1713 = String To Path(string=w1767) -> (path=w1775:path)
            n1714 = String To Path(string=w1766) -> (path=w1774:path)
            n1715 = String To Path(string=w1765) -> (path=w1773:path)
            n1716 = case shown="True" w1764 {
              tunnel: [w1780 w1781] -> w1768
              frame False {
                n1717 = local read "string1"() -> (w1780:string)
              }
              frame True {
                n1718 = local read "String Indicator 4"() -> (w1781:string)
              }
            }
            n1719 = Open/Create/Replace File "Open File"(file path (use dialog)=w1775) -> (refnum out=w1771:refnum<file>)  [unwired: 5 in, 2 out]
            n1720 = Open/Create/Replace File "Open File"(file path (use dialog)=w1774) -> (refnum out=w1770:refnum<file>)  [unwired: 5 in, 2 out]
            n1721 = Open/Create/Replace File "Open File"(file path (use dialog)=w1773) -> (refnum out=w1769:refnum<file>)  [unwired: 5 in, 2 out]
            n1722 = while {
              tunnel: w1771 -> [w1793]
              i -> [w1789]
              stop <- w1788 continue-if-true
              (unwired) TRUE ("line mode (F)")
              n1723 = Read from Text File "Read File"(file (use dialog)=w1793) -> (text=w1790:string)  [unwired: 3 in, 3 out]
              n1724 = local write "Numeric 11"(w1789) -> ()
              n1725 = String Length(string=w1790) -> (length=w1792:i32)
              n1726 = Greater?(x=w1792, y=1) -> (0:w1788:bool)
            }
            n1727 = while {
              tunnel: w1770 -> [w1799]
              i -> [w1795]
              stop <- w1794 continue-if-true
              (unwired) TRUE ("line mode (F)")
              n1728 = Read from Text File "Read File"(file (use dialog)=w1799) -> (text=w1796:string)  [unwired: 3 in, 3 out]
              n1729 = local write "Numeric 12"(w1795) -> ()
              n1730 = String Length(string=w1796) -> (length=w1798:i32)
              n1731 = Greater?(x=w1798, y=1) -> (0:w1794:bool)
            }
            n1732 = while {
              tunnel: w1769 -> [w1805]
              i -> [w1801]
              stop <- w1800 continue-if-true
              (unwired) TRUE ("line mode (F)")
              n1733 = Read from Text File "Read File"(file (use dialog)=w1805) -> (text=w1802:string)  [unwired: 3 in, 3 out]
              n1734 = local write "Numeric 13"(w1801) -> ()
              n1735 = String Length(string=w1802) -> (length=w1804:i32)
              n1736 = Greater?(x=w1804, y=1) -> (0:w1800:bool)
            }
            n1737 = String To Path(string=w1768) -> (path=w1776:path)
            n1738 = Open/Create/Replace File "Open File"(file path (use dialog)=w1776) -> (refnum out=w1772:refnum<file>)  [unwired: 5 in, 2 out]
            n1739 = while {
              tunnel: w1772 -> [w1787]
              i -> [w1783]
              stop <- w1782 continue-if-true
              (unwired) TRUE ("line mode (F)")
              n1740 = Read from Text File "Read File"(file (use dialog)=w1787) -> (text=w1784:string)  [unwired: 3 in, 3 out]
              n1741 = local write "Numeric 8"(w1783) -> ()
              n1742 = String Length(string=w1784) -> (length=w1786:i32)
              n1743 = Greater?(x=w1786, y=1) -> (0:w1782:bool)
            }
          }
          frame #1 {
            w1957 = FALSE ("ACTUAL   MERGE")
            # "Sample Temp"
            # "ECR"
            # "COF"
            # "Time\nCOF\nFF\nTemp"
            n1744 = case shown="True" w1830 {
              tunnel: [w1977 w1978] -> w1831
              frame False {
                n1745 = local read "string1"() -> (w1977:string)
              }
              frame True {
                n1746 = local read "String Indicator 4"() -> (w1978:string)
              }
            }
            n1747 = local read "string1 3"() -> (w1875:string)
            n1748 = String To Path(string=w1831) -> (path=w1962:path)
            n1749 = String To Path(string=w1875) -> (path=w1973:path)
            n1750 = local read "Numeric 12"() -> (w1959:i32)
            n1751 = local read "Numeric 8"() -> (w1961:i32)
            n1752 = local read "string1 2"() -> (w1876:string)
            n1753 = local read "string1 4"() -> (w1874:string)
            n1754 = Open/Create/Replace File "Open File"(file path (use dialog)=w1962) -> (refnum out=w1976:refnum<file>, error out=w1975:errorcluster)  [unwired: 5 in, 1 out]
            n1755 = Open/Create/Replace File "Open File"(file path (use dialog)=w1973) -> (refnum out=w1969:refnum<file>, error out=w1970:errorcluster)  [unwired: 5 in, 1 out]
            n1756 = for {
              N: w1961 -> [_]
              tunnel: w1976 -> [w2124]
              tunnel: w1975 -> [w2123]
              tunnel: [w2113] -> w1888 mode=indexing
              tunnel: [w2111] -> w1945 mode=indexing
              tunnel: [w2112] -> w1940 mode=indexing
              tunnel: w1957 -> [_]
              tunnel: [w2105] -> w1942 mode=indexing
              tunnel: [w2101] -> w1911 mode=indexing
              tunnel: [w2097] -> w1886 mode=indexing
              tunnel: [w2093] -> w1867 mode=indexing
              tunnel: [w2088] -> w1827 mode=indexing
              (unwired) TRUE ("line mode (F)")
              # "freq"
              # "Stroke"
              # "Time"
              # "CoF"
              # "Humidity"
              # "Temp"
              # "Air Temp"
              # "ECR"
              n1757 = Read from Text File "Read File"(file (use dialog)=w2124, error in=w2123) -> (text=w2089:string)  [unwired: 2 in, 3 out]
              n1758 = local write "String 6"(w2089) -> ()
              n1759 = String Subset(string=w2089, offset (0)=0, length (rest)=14 ("length (rest)")) -> (substring=w2117:string)
              n1760 = String Subset(string=w2089, offset (0)=35, length (rest)=9 ("length (rest)")) -> (substring=w2114:string)
              n1761 = String Subset(string=w2089, offset (0)=15, length (rest)=9 ("length (rest)")) -> (substring=w2120:string)
              n1762 = Fract/Exp String To Number(string=w2117) -> (number=w2113:dbl)  [unwired: 3 in, 1 out]
              n1763 = Fract/Exp String To Number(string=w2114) -> (number=w2112:dbl)  [unwired: 3 in, 1 out]
              n1764 = Fract/Exp String To Number(string=w2120) -> (number=w2111:dbl)  [unwired: 3 in, 1 out]
              n1765 = String Subset(string=w2089, offset (0)=85, length (rest)=9 ("length (rest)")) -> (substring=w2090:string)
              n1766 = String Subset(string=w2089, offset (0)=25, length (rest)=9 ("length (rest)")) -> (substring=w2096:string)
              n1767 = String Subset(string=w2089, offset (0)=55, length (rest)=9 ("length (rest)")) -> (substring=w2098:string)
              n1768 = String Subset(string=w2089, offset (0)=45, length (rest)=9 ("length (rest)")) -> (substring=w2104:string)
              n1769 = String Subset(string=w2089, offset (0)=65, length (rest)=9 ("length (rest)")) -> (substring=w2110:string)
              n1770 = Fract/Exp String To Number(string=w2096) -> (number=w2093:dbl)  [unwired: 3 in, 1 out]
              n1771 = Fract/Exp String To Number(string=w2090) -> (number=w2088:dbl)  [unwired: 3 in, 1 out]
              n1772 = Fract/Exp String To Number(string=w2098) -> (number=w2097:dbl)  [unwired: 3 in, 1 out]
              n1773 = Fract/Exp String To Number(string=w2104) -> (number=w2101:dbl)  [unwired: 3 in, 1 out]
              n1774 = Fract/Exp String To Number(string=w2110) -> (number=w2107:dbl)  [unwired: 3 in, 1 out]
              n1775 = Add(x=w2107, y=0.0) -> (x+y=w2105:dbl)
            }
            n1776 = for {
              N: w1959 -> [_]
              tunnel: w1970 -> [w2050]
              tunnel: w1969 -> [w2049]
              tunnel: [w2039] -> w1928 mode=indexing
              tunnel: [w2037] -> w1926 mode=indexing
              tunnel: [w2038] -> w1922 mode=indexing
              tunnel: w1957 -> [_]
              tunnel: [w2031] -> w1924 mode=indexing
              tunnel: [w2027] -> w1906 mode=indexing
              tunnel: [w2023] -> w1882 mode=indexing
              tunnel: [w2020] -> w1863 mode=indexing
              tunnel: [w2016] -> w1822 mode=indexing
              (unwired) 9 ("length (rest)")
              (unwired) 9 ("length (rest)")
              (unwired) TRUE ("line mode (F)")
              n1777 = Read from Text File "Read File"(file (use dialog)=w2049, error in=w2050) -> (text=w2017:string)  [unwired: 2 in, 3 out]
              n1778 = local write "String 8"(w2017) -> ()
              n1779 = String Subset(string=w2017, offset (0)=85) -> (substring=w2019:string)  [unwired: 1 in]
              n1780 = String Subset(string=w2017, offset (0)=35, length (rest)=9 ("length (rest)")) -> (substring=w2040:string)
              n1781 = String Subset(string=w2017, offset (0)=55, length (rest)=9 ("length (rest)")) -> (substring=w2025:string)
              n1782 = String Subset(string=w2017, offset (0)=25) -> (substring=w2021:string)  [unwired: 1 in]
              n1783 = String Subset(string=w2017, offset (0)=15, length (rest)=9 ("length (rest)")) -> (substring=w2046:string)
              n1784 = String Subset(string=w2017, offset (0)=0, length (rest)=14 ("length (rest)")) -> (substring=w2043:string)
              n1785 = String Subset(string=w2017, offset (0)=45, length (rest)=9 ("length (rest)")) -> (substring=w2030:string)
              n1786 = String Subset(string=w2017, offset (0)=65, length (rest)=9 ("length (rest)")) -> (substring=w2036:string)
              n1787 = Fract/Exp String To Number(string=w2019) -> (number=w2016:dbl)  [unwired: 3 in, 1 out]
              n1788 = Fract/Exp String To Number(string=w2040) -> (number=w2038:dbl)  [unwired: 3 in, 1 out]
              n1789 = Fract/Exp String To Number(string=w2025) -> (number=w2023:dbl)  [unwired: 3 in, 1 out]
              n1790 = Fract/Exp String To Number(string=w2021) -> (number=w2020:dbl)  [unwired: 3 in, 1 out]
              n1791 = Fract/Exp String To Number(string=w2046) -> (number=w2037:dbl)  [unwired: 3 in, 1 out]
              n1792 = Fract/Exp String To Number(string=w2043) -> (number=w2039:dbl)  [unwired: 3 in, 1 out]
              n1793 = Fract/Exp String To Number(string=w2030) -> (number=w2027:dbl)  [unwired: 3 in, 1 out]
              n1794 = Fract/Exp String To Number(string=w2036) -> (number=w2033:dbl)  [unwired: 3 in, 1 out]
              n1795 = Add(x=w2033, y=0.0) -> (x+y=w2031:dbl)
            }
            n1796 = String To Path(string=w1876) -> (path=w1974:path)
            n1797 = String To Path(string=w1874) -> (path=w1968:path)
            n1798 = local read "Numeric 11"() -> (w1958:i32)
            n1799 = local read "Numeric 13"() -> (w1960:i32)
            n1800 = Open/Create/Replace File "Open File"(file path (use dialog)=w1974) -> (refnum out=w1972:refnum<file>, error out=w1971:errorcluster)  [unwired: 5 in, 1 out]
            n1801 = Open/Create/Replace File "Open File"(file path (use dialog)=w1968) -> (refnum out=w1967:refnum<file>, error out=w1966:errorcluster)  [unwired: 5 in, 1 out]
            n1802 = for {
              N: w1958 -> [_]
              tunnel: w1972 -> [w2087]
              tunnel: w1971 -> [w2086]
              tunnel: [w2076] -> w1938 mode=indexing
              tunnel: [w2074] -> w1936 mode=indexing
              tunnel: [w2075] -> w1931 mode=indexing
              tunnel: w1957 -> [_]
              tunnel: [w2068] -> w1933 mode=indexing
              tunnel: [w2064] -> w1909 mode=indexing
              tunnel: [w2060] -> w1884 mode=indexing
              tunnel: [w2056] -> w1865 mode=indexing
              tunnel: [w2051] -> w1823 mode=indexing
              (unwired) TRUE ("line mode (F)")
              n1803 = Read from Text File "Read File"(file (use dialog)=w2087, error in=w2086) -> (text=w2052:string)  [unwired: 2 in, 3 out]
              n1804 = local write "String 7"(w2052) -> ()
              n1805 = String Subset(string=w2052, offset (0)=85, length (rest)=9 ("length (rest)")) -> (substring=w2055:string)
              n1806 = String Subset(string=w2052, offset (0)=35, length (rest)=9 ("length (rest)")) -> (substring=w2077:string)
              n1807 = String Subset(string=w2052, offset (0)=55, length (rest)=9 ("length (rest)")) -> (substring=w2063:string)
